vi "Find Overlapping Area.vi"(8 "Error In":errorcluster, 11 "List of Trimmed Claims":string[](array[string])=["1,3,4,4", "3,1,4,4", "5,5,2,2"]) -> (0 "Error Out":errorcluster, 2 "Fabric Claims":T1, 3 "in^2 of Overlapping Claims":i32)   [LabVIEW 2019]
doc: "Given a list (1d string array) of trimmed claims (\"A,B,C,D\" where A is the distance in inches from the left edge, B is the distance in inches from the top edge, C is the width of the claim, and D is the height of the claim), output the total number of square inches that have been claimed multiple times. \n\nOptionally, this also outputs the whole fabric map with the number of claims for each square inch.\n\nNote: this will only work for integer claims."
uses:
  <vilib>/silver_ctls/ArrayMatrixCluster/Real Matrix NI_Silver.ctl
  <vilib>/Analysis/Matrix/Datatypes/RealMatrix.ctl
  <vilib>/Analysis/Matrix/Numeric/Add/Add - RM,RM.vi
  <vilib>/Analysis/Matrix/Numeric/Conversions/Matrix To Array - RM.vi
  <vilib>/Analysis/Matrix/NI_Matrix.lvlib
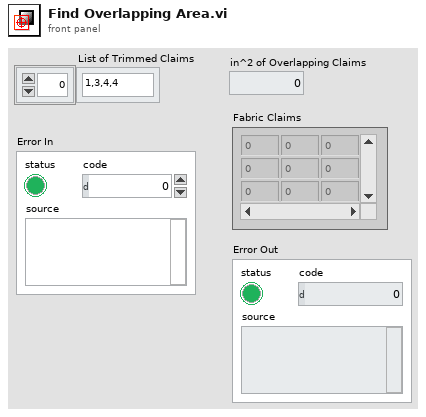
[diagram p1: front panel]
types:
  T1 = typedef "Real Matrix NI_Silver.ctl" = dbl[][]
  T2 = typedef "NI_Matrix.lvlib/RealMatrix.ctl" = dbl[][]
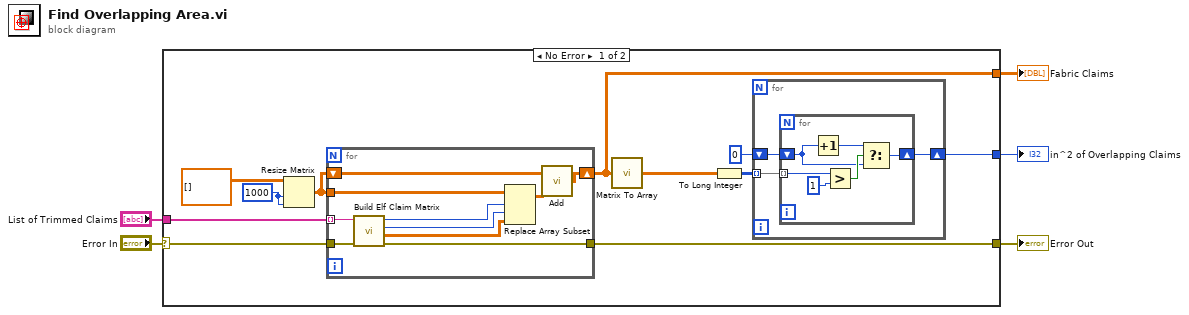
[diagram p0: block diagram]
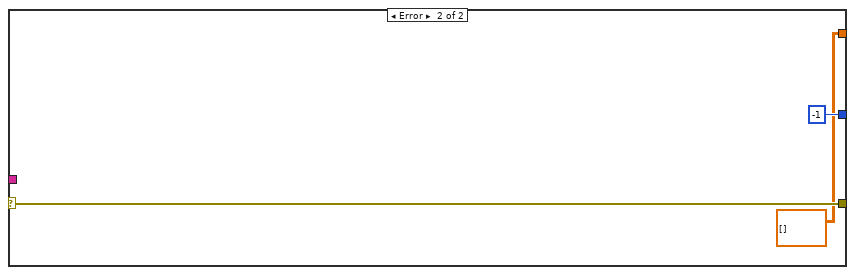
[diagram p2: hidden frame]
diagram:
  n1 = case shown="No Error" "Error In" {
    selector: "Error In" -> [w7 w38]
    tunnel: "List of Trimmed Claims" -> [w12 _]
    tunnel: [w9 -1] -> w4
    tunnel: [w6 w38] -> w2
    tunnel: [w8 T2 [] ("matrix")] -> w1
    frame No Error {
      w11 = 1000 ("number of rows")
      n2 = Resize Matrix(1:w11, 2:w11, 4:T2 [] ("matrix")) -> (0:w16:T2)
      n3 = for {
        tunnel: w12 -> [w28] mode=indexing
        shift-right: [w30] -> w8
        shift-left: w16 -> [w32]
        tunnel: w16 -> [w35]
        tunnel: w7 -> [w27]
        tunnel: [w26] -> w6
        n4 = call "Build Elf Claim Matrix.vi"("Error In"=w27, "Elf Claim"=w28) -> ("Error Out"=w26:errorcluster, "Elf Claim Matrix"=w29:T1, "Distance from Top Edge"=w33:i32, "Distance from Left Edge"=w34:i32)  [unwired: 4 in, 2 out]
        n5 = Replace Array Subset(array=w35, new element=w29, index (row)=w34, index (col)=w33) -> (w31:T2)
        n6 = call-poly <vilib>:"Add.vi"("Real Matrix B"=w31, "Real Matrix A"=w32) -> ("A + B"=w30:T2)
      }
      n7 = call-poly <vilib>:"Matrix To Array.vi"("Real Matrix"=w8) -> ("Real 2D Array"=w15:dbl[][])
      n8 = To Long Integer(number=w15) -> (32bit integer=w14:i32[][])
      n9 = for {
        tunnel: w14 -> [w19] mode=indexing
        shift-right: [w17] -> w9
        shift-left: 0 -> [w18]
        n10 = for {
          tunnel: w19 -> [w24] mode=indexing
          shift-right: [w20] -> w17
          shift-left: w18 -> [w21]
          n11 = Increment(x=w21) -> (x+1=w22:i32)
          n12 = Greater?(x=w24, y=1) -> (0:w23:bool)
          n13 = Select(t=w22, s=w23, f=w21) -> (s? t:f=w20:i32)
        }
      }
    }
    frame Error {
    }
  }
  "in^2 of Overlapping Claims" <- w4
  "Error Out" <- w2
  "Fabric Claims" <- w1
